vi "ItalicTag.vi"(8 "error in (no error)":errorcluster, 11 "Bold in":refnum<class "Italic.lvclass">) -> (0 "error out":errorcluster, 2 "BoldTag":string, 3 "Bold out":refnum<class "Italic.lvclass">)   [LabVIEW 2021, in "LvMarkdown.lvlib" / "Italic.lvclass"]
uses:
  Italic.lvclass
  Italic.lvclass/Italic.ctl
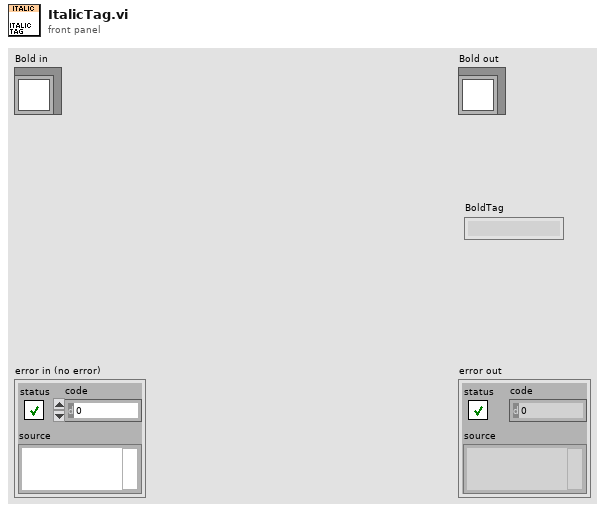
[diagram p1: front panel]
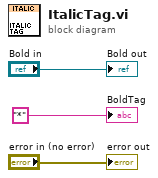
[diagram p0: block diagram]
diagram:
  "error out" <- "error in (no error)"
  "Bold out" <- "Bold in"
  "BoldTag" <- "*" ("BoldTag")
